vi "Wczytanie_ustawien_Rej.vi"(8 "error in (no error)":errorcluster, 11 "Plik konf in":path=path "D:/Marek/Dysk Google/Projekty LabVIEW/! Rudpol/Program/Konfiguracja/AI_Konfiguracja.txt") -> (0 "error out":errorcluster, 2 "Rej_konfig_out":T2[](array[typedef]) {"Wolna Wykr num" items=["Brak", "Wykres 1", "Wykres 2", "Wykres 3", "Wykres 4"]}, 3 "Plik konf out":path)   [LabVIEW 2013]
doc: "Use this template to build a VI to use as a subVI."
uses:
  Kontrolki/GUI/RejWol_konfig.ctl
  Kontrolki/GUI/RejWol_typ.ctl
  Kontrolki/GUI/Wolna_WykrNum.ctl
panel:
  out "*(type *) &x":T1
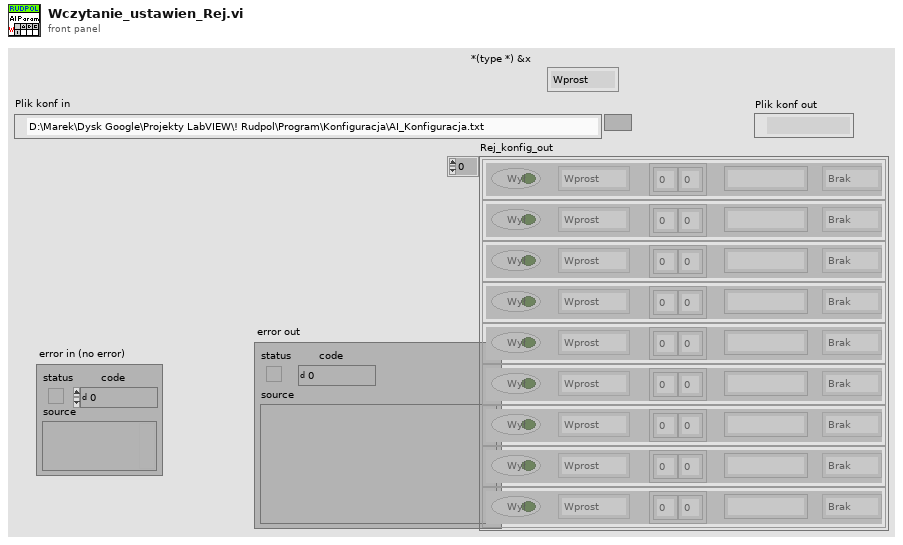
[diagram p1: front panel]
types:
  T1 = typedef "RejWol_typ.ctl" = enum16{"Wprost", "Moduł", "Kwadrat", "Iloczyn", "Faza"}
  T2 = typedef "RejWol_konfig.ctl" = cluster{"Typ rejestracji":T1, "Kanały":i32[], "Opis":string, "Aktywny":bool, "Wolna Wykr num":T3}
  T3 = typedef "Wolna_WykrNum.ctl" = u16
  T4 = enum16{"open", "replace", "create", "open or create", "replace or create", "replace or create with confirmation"}
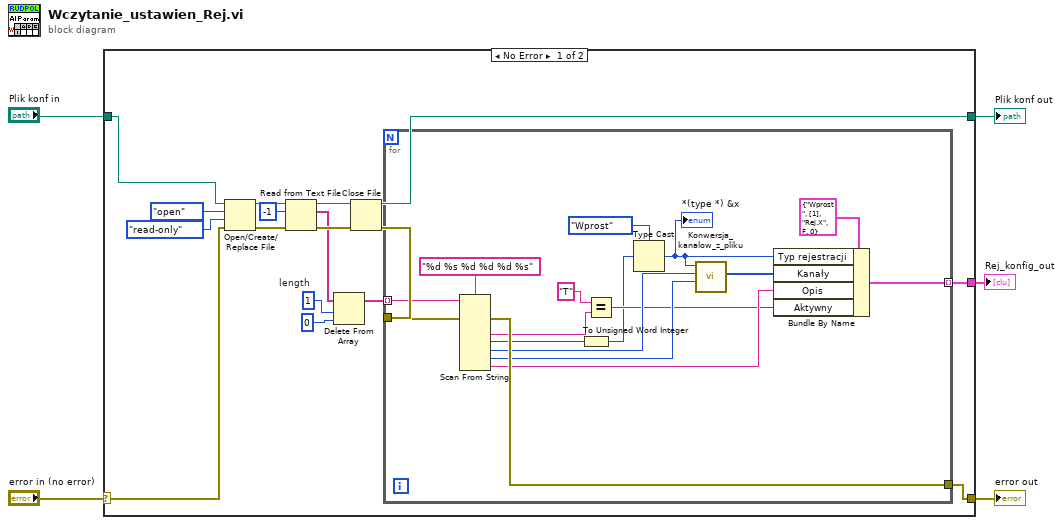
[diagram p0: block diagram]
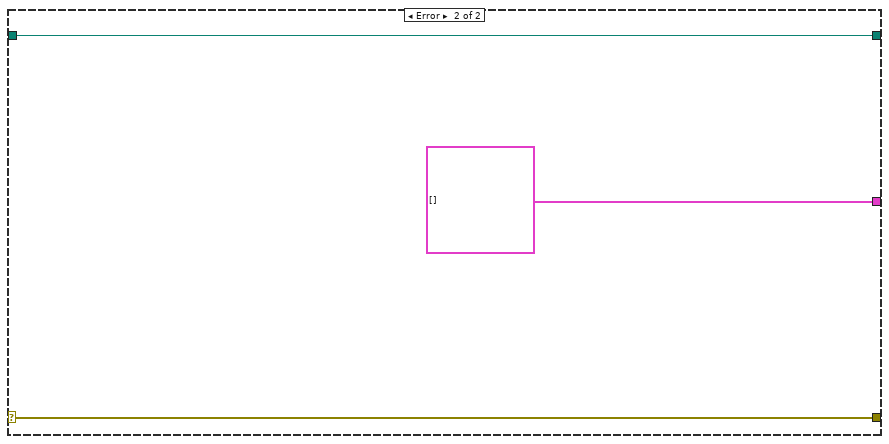
[diagram p2: hidden frame]
diagram:
  n1 = case shown="No Error" "error in (no error)" {
    selector: "error in (no error)" -> [w10 w42]
    tunnel: [w9 w42] -> w4
    tunnel: "Plik konf in" -> [w15 w41]
    tunnel: [w14 w41] -> w3
    tunnel: [w7 T2[] [] ("Rej_konfig_out")] -> w1
    frame No Error {
      w12 = 1  # length
      n2 = Open/Create/Replace File(file path (use dialog)=w15, error in=w10, operation (0:open)=T4."open", access (0:read/write)=enum16{"read/write", "read-only", "write-only"}."read-only") -> (refnum out=w19:refnum<file>, error out=w20:errorcluster)  [unwired: 2 in, 1 out]
      n3 = Read from Text File(file (use dialog)=w19, count=-1, error in=w20) -> (refnum out=w17:refnum<file>, text=w8:string[], error out=w18:errorcluster)  [unwired: 1 in, 1 out]
      n4 = Delete From Array(array=w8, length=w12, index=0) -> (array with subset deleted=w6:string[])  [unwired: 1 out]
      n5 = Close File(refnum=w17, error in=w18) -> (path=w14:path, error out=w11:errorcluster)
      n6 = for {
        tunnel: w6 -> [w39] mode=indexing
        tunnel: w11 -> [w38]
        tunnel: [w37] -> w9
        tunnel: [w26] -> w7 mode=indexing
        n7 = Scan From String(format string="%d %s %d %d %d %s", input string=w39, error in=w38) -> (error out=w37:errorcluster, output 2=w29:string, output 3=w23:i32, output 4=w32:i32, output 5=w31:i32, output 6=w30:string)  [unwired: 8 in, 2 out]
        n8 = To Unsigned Word Integer(number=w23) -> (unsigned 16bit integer=w24:u16)
        n9 = Equal?(x="T", y=w29) -> (x = y?=w27:bool)
        n10 = Type Cast(type=RejWol_typ."Wprost" ("Typ rejestracji"), x=w24) -> (*(type *) &x=w33:T1)
        "*(type *) &x" <- w33
        n11 = call "Konwersja_kanalow_z_pliku.vi"("Kanal 2"=w31, "Kanal 1"=w32, "Typ rejestracji"=w33) -> ("Kanaly"=w25:i32[])  [unwired: 8 in]
        n12 = Bundle By Name(cluster=T2 {"Typ rejestracji"=enum."Wprost", "Kanały"=[1], "Opis"="Rej.X", "Aktywny"=FALSE, "Wolna Wykr num"=0} ("Rejestracja AI"), "Typ rejestracji"=w33, "Kanały"=w25, "Opis"=w30, "Aktywny"=w27) -> (w26:T2)
      }
    }
    frame Error {
    }
  }
  "error out" <- w4
  "Plik konf out" <- w3
  "Rej_konfig_out" <- w1
